vi "Logging Engine.vi"() -> ()   [LabVIEW 2016]
uses:
  <vilib>/DAQmx/read.llb/DAQmx Read (Analog Wfm 1Chan NSamp).vi
  <vilib>/TagLibrary/Create Tag (Int).vi
  <vilib>/TagLibrary/Write (Int).vi
  <vilib>/TagLibrary/Create Tag (String).vi
  <vilib>/TagLibrary/Write (String).vi
  <vilib>/TagLibrary/Write (Double).vi
  <vilib>/Message/Open (Sync).vi
  <vilib>/Message/Subscribe (Sync).vi
  <vilib>/DAQmx/miscellaneous.llb/DAQmx Fill In Error Info.vi
  <vilib>/Waveform/WDTOps.llb/WDT Number of Waveform Samples DBL.vi
  <vilib>/Waveform/WDTOps.llb/WDT Append Waveforms DBL.vi
  <vilib>/Message/Publish (Sync).vi
  <vilib>/TagLibrary/Read (Double).vi
  <vilib>/DAQmx/configure/timing.llb/DAQmx Timing (Sample Clock).vi
  <vilib>/TagLibrary/Read (Int).vi
  <vilib>/TagLibrary/Read (String).vi
  <vilib>/DAQmx/create/channels.llb/DAQmx Create Channel (AI-Temperature-Thermocouple).vi
  <vilib>/TagLibrary/Tag Library.lvlib
  <resource>/objmgr/niTag.rc
  <resource>/objmgr/daqmx.rc
panel:
  in  "Acquiring":bool
  out "Send Time":timestamp
  in  "Log":bool
  out "Status":string
  out "Channel":string
  out "error out":errorcluster
  out "Iteration":i32
  out "Waveform Channel":string
  in  "Send File":bool
  out "Sample Rate":dbl=1000.0 format="%0.2f"
  out "Files Sent":i32
  out "Buffered":i32
  in  "stop":bool
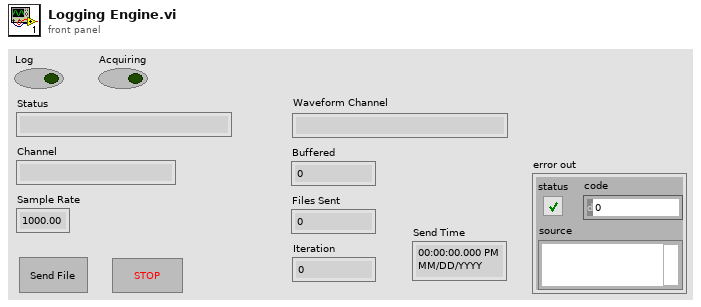
[diagram p1: front panel]
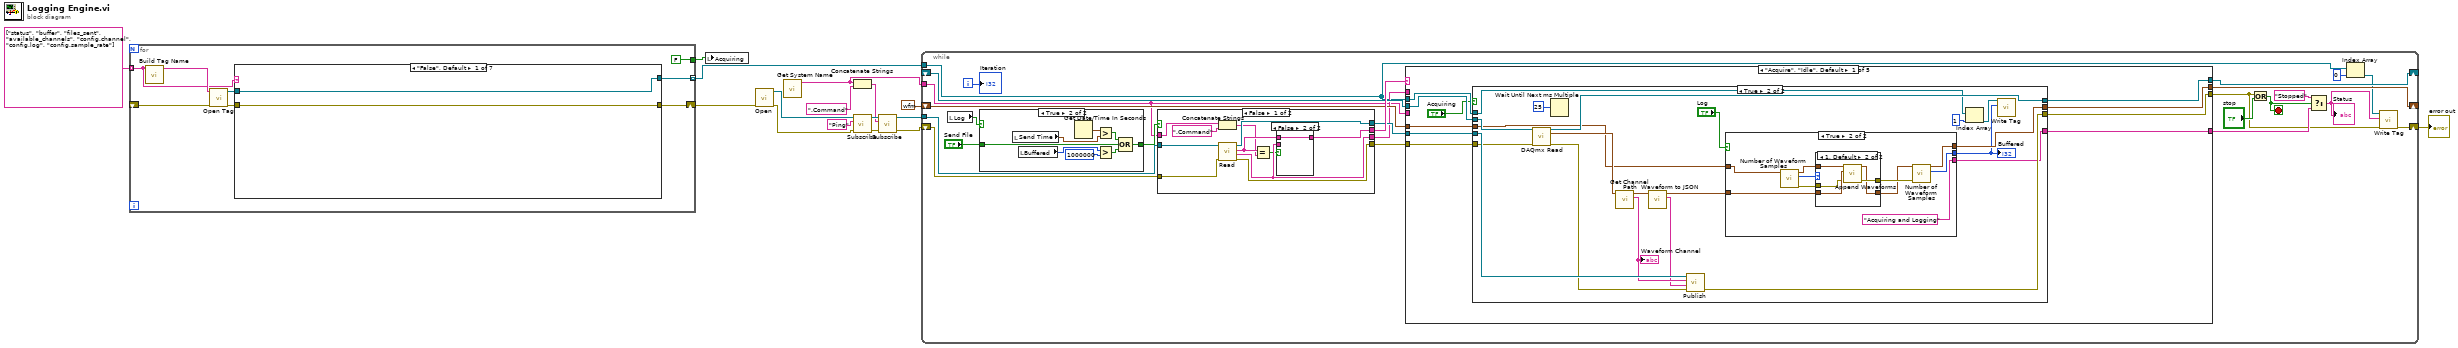
[diagram p0: block diagram]
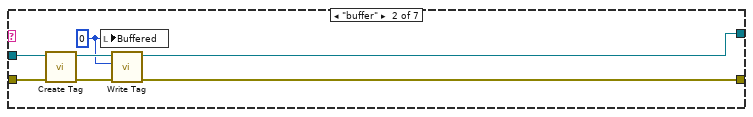
[diagram p2: hidden frame]
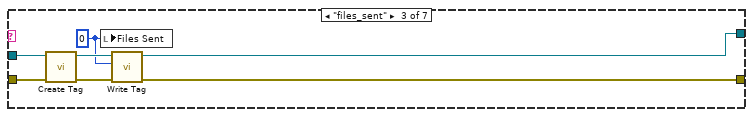
[diagram p3: hidden frame]
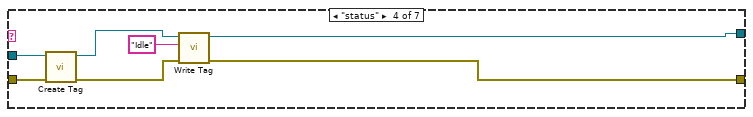
[diagram p4: hidden frame]
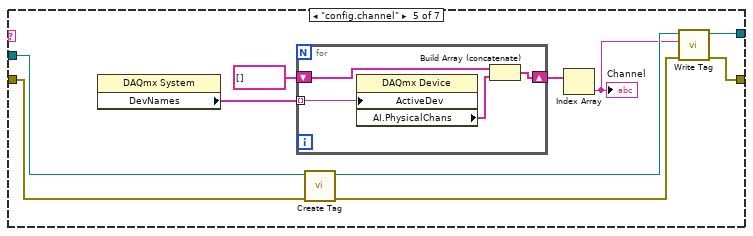
[diagram p5: hidden frame]
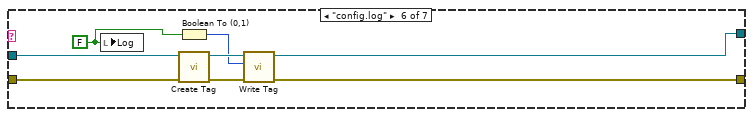
[diagram p6: hidden frame]
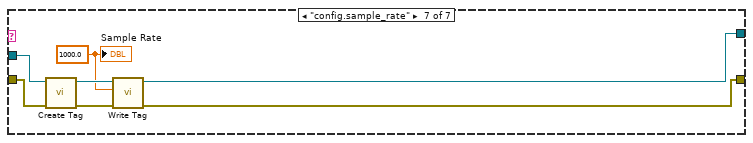
[diagram p7: hidden frame]
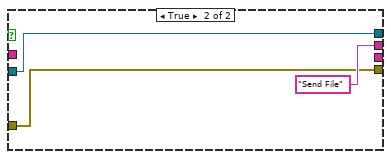
[diagram p10: hidden frame]
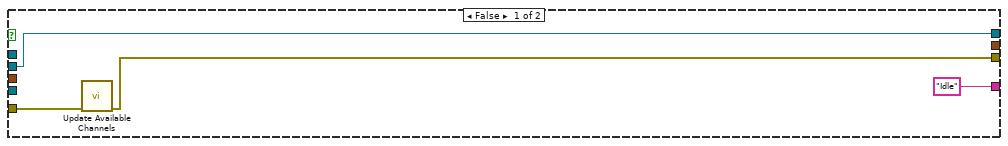
[diagram p11: hidden frame]
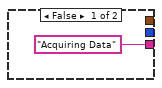
[diagram p12: hidden frame]
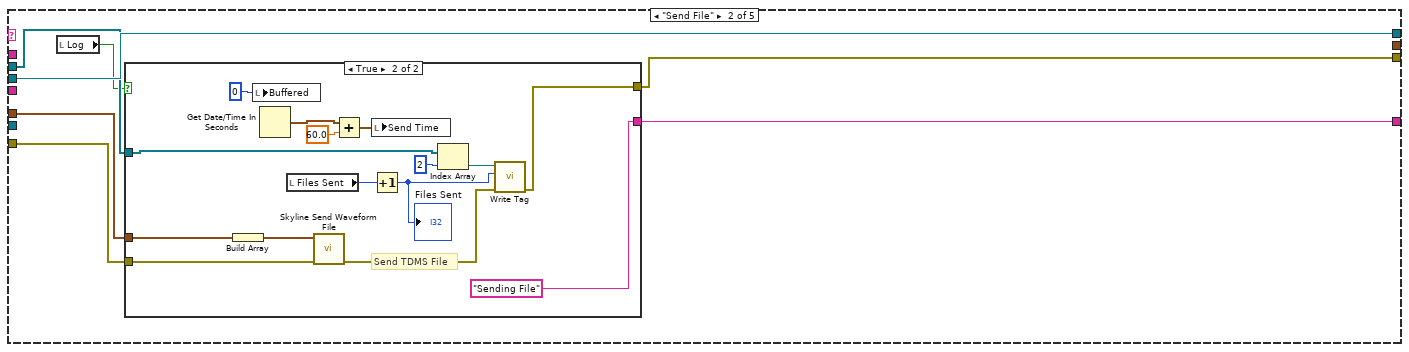
[diagram p14: hidden frame]
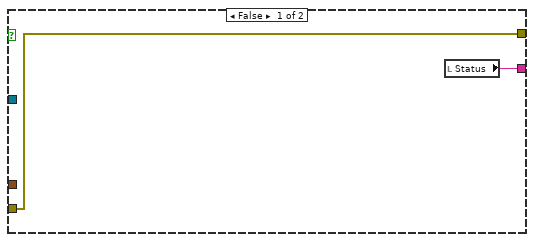
[diagram p15: hidden frame]
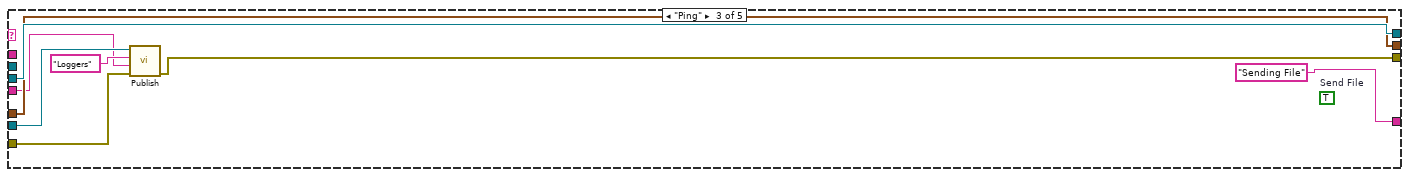
[diagram p16: hidden frame]
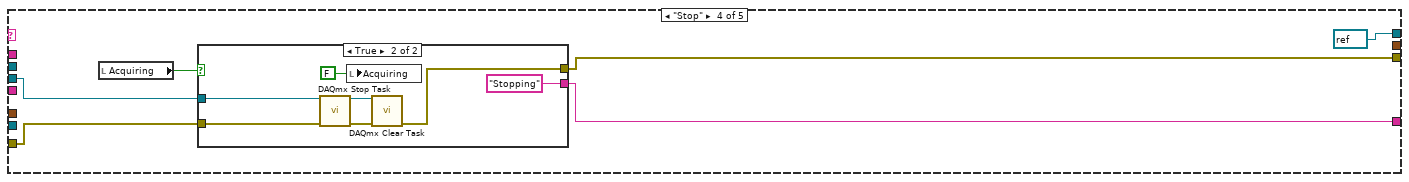
[diagram p17: hidden frame]
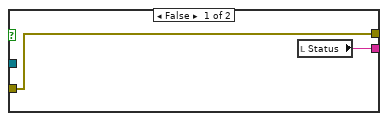
[diagram p18: hidden frame]
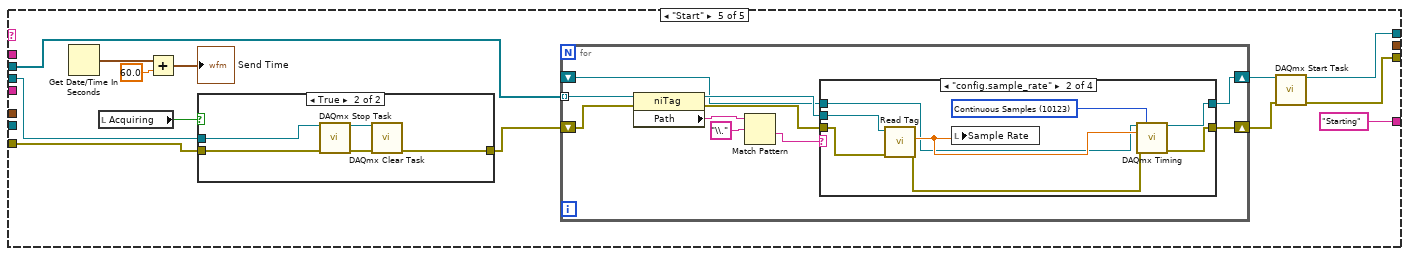
[diagram p19: hidden frame]
diagram:
  n1 = for {
    tunnel: [w23] -> w16 mode=indexing
    tunnel: string[] ["status", "buffer", "files_sent", "available_channels", "config.channel", "config.log", "config.sample_rate"] -> [w20] mode=indexing
    shift-right: [w19] -> w4
    shift-left: _ -> [w18]
    tunnel: [FALSE ("Acquiring")] -> w2
    n2 = call "Build Tag Name.vi"("Tag"=w20) -> ("System Tag"=w24:string)  [unwired: 10 in]
    n3 = call <vilib>:"Open Tag.vi"("error in (no error)"=w18, "tag path"=w24) -> ("error out"=w21:errorcluster, "tag reference out"=w22:refnum<k21>)  [unwired: 8 in]
    n4 = case shown="\"False\", Default" w20 {
      tunnel: [w25 w31 w38 w45 w53 w65 w72] -> w23
      tunnel: w22 -> [w25 w30 w37 w44 w57 w69 w76]
      tunnel: w21 -> [w26 w29 w36 w43 w56 w68 w75]
      tunnel: [w26 w28 w35 w41 w54 w66 w73] -> w19
      frame "False", Default {
      }
      frame "buffer" {
        w27 = 0 ("y")
        n5 = call-poly <vilib>:"Create Tag.vi"("error in (no error)"=w29, "tag reference in"=w30) -> ("error out"=w33:errorcluster, "tag reference out"=w32:refnum<k21>)  [unwired: 8 in]
        n6 = local write "Buffered"(w27) -> ()
        n7 = call-poly <vilib>:"Write Tag.vi"("error in (no error)"=w33, "int"=w27, "tag reference in"=w32) -> ("error out"=w28:errorcluster, "tag reference out"=w31:refnum<k21>)  [unwired: 7 in]
      }
      frame "files_sent" {
        w34 = 0 ("y")
        n8 = call-poly <vilib>:"Create Tag.vi"("error in (no error)"=w36, "tag reference in"=w37) -> ("error out"=w40:errorcluster, "tag reference out"=w39:refnum<k21>)  [unwired: 8 in]
        n9 = local write "Files Sent"(w34) -> ()
        n10 = call-poly <vilib>:"Write Tag.vi"("error in (no error)"=w40, "int"=w34, "tag reference in"=w39) -> ("error out"=w35:errorcluster, "tag reference out"=w38:refnum<k21>)  [unwired: 7 in]
      }
      frame "status" {
        n11 = call-poly <vilib>:"Create Tag.vi"("error in (no error)"=w43, "tag reference in"=w44) -> ("error out"=w47:errorcluster, "tag reference out"=w46:refnum<k21>)  [unwired: 8 in]
        n12 = call-poly <vilib>:"Write Tag.vi"("error in (no error)"=w47, "string"="Idle", "tag reference in"=w46) -> ("error out"=w41:errorcluster, "tag reference out"=w45:refnum<k21>)  [unwired: 7 in]
      }
      frame "config.channel" {
        n13 = property class="DAQmx System"() -> ("DevNames"=w51:tag[])  [unwired: 2 in, 2 out]
        n14 = for {
          tunnel: w51 -> [w61] mode=indexing
          shift-right: [w59] -> w49
          shift-left: string[] [] -> [w60]
          n15 = property class="DAQmx Device"("ActiveDev"=w61) -> ("AI.PhysicalChans"=w58:tag[])  [unwired: 2 in, 2 out]
          n16 = Build Array (concatenate)(w60, w58) -> (w59:string[])
        }
        n17 = call-poly <vilib>:"Create Tag.vi"("error in (no error)"=w56, "tag reference in"=w57) -> ("error out"=w52:errorcluster, "tag reference out"=w55:refnum<k21>)  [unwired: 8 in]
        n18 = Index Array(array=w49) -> (element=w48:string)  [unwired: 1 in]
        "Channel" <- w48
        n19 = call-poly <vilib>:"Write Tag.vi"("error in (no error)"=w52, "string"=w48, "tag reference in"=w55) -> ("error out"=w54:errorcluster, "tag reference out"=w53:refnum<k21>)  [unwired: 7 in]
      }
      frame "config.log" {
        w62 = FALSE ("Log")
        n20 = local write "Log"(w62) -> ()
        n21 = Boolean To (0,1)(Boolean=w62) -> (0, 1=w63:i16)
        n22 = call-poly <vilib>:"Create Tag.vi"("error in (no error)"=w68, "tag reference in"=w69) -> ("error out"=w64:errorcluster, "tag reference out"=w67:refnum<k21>)  [unwired: 8 in]
        n23 = call-poly <vilib>:"Write Tag.vi"("error in (no error)"=w64, "int"=w63, "tag reference in"=w67) -> ("error out"=w66:errorcluster, "tag reference out"=w65:refnum<k21>)  [unwired: 7 in]
      }
      frame "config.sample_rate" {
        w70 = 1000.0 ("double")
        n24 = call-poly <vilib>:"Create Tag.vi"("error in (no error)"=w75, "tag reference in"=w76) -> ("error out"=w71:errorcluster, "tag reference out"=w74:refnum<k21>)  [unwired: 8 in]
        n25 = call-poly <vilib>:"Write Tag.vi"("error in (no error)"=w71, "double"=w70, "tag reference in"=w74) -> ("error out"=w73:errorcluster, "tag reference out"=w72:refnum<k21>)  [unwired: 7 in]
        "Sample Rate" <- w70
      }
    }
  }
  n26 = local write "Acquiring"(w2) -> ()
  n27 = call-poly <vilib>:"Open.vi"("error in"=w4) -> ("error out"=w8:errorcluster, "Message Sync Refnum"=w9:refnum<k21>)  [unwired: 9 in]
  n28 = call "Get System Name.vi"() -> ("System Name"=w7:string)  [unwired: 11 in]
  n29 = Concatenate Strings(w7, ".Command" ("topic")) -> (w5:string)
  n30 = call-poly <vilib>:"Subscribe.vi"("error in (no error)"=w8, "topic"="Ping", "Message Sync Refnum"=w9) -> ("error out"=w11:errorcluster, "Message Sync Refnum"=w10:refnum<k21>)  [unwired: 7 in]
  n31 = call-poly <vilib>:"Subscribe.vi"("error in (no error)"=w11, "topic"=w5, "Message Sync Refnum"=w10) -> ("error out"=w13:errorcluster, "Message Sync Refnum"=w14:refnum<k21>)  [unwired: 7 in]
  n32 = while {
    shift-right: [w91] -> _
    shift-left: waveform(dbl) {"t0"=timestamp(0 s since 1904-01-01), "dt"=1.0, "Y"=[]} ("Waveform") -> [w93]
    tunnel: w16 -> [w89]
    tunnel: w14 -> [w97]
    shift-right: [w99] -> _
    shift-left: _ -> [w98]
    shift-right: [w81] -> w3
    shift-left: w13 -> [w96]
    tunnel: w7 -> [w86]
    i -> [w101]
    stop <- w84 stop-if-true
    n33 = local read "Log"() -> (w78:bool)
    n34 = case shown="True" w78 {
      tunnel: [_ w109] -> w90
      tunnel: "Send File" -> [_ w102]
      frame False {
      }
      frame True {
        n35 = local read "Send Time"() -> (w107:timestamp)
        n36 = local read "Buffered"() -> (w105:i32)
        n37 = Get Date/Time In Seconds() -> (seconds since 1Jan1904=w108:timestamp)
        n38 = Greater?(x=w108, y=w107) -> (0:w106:bool)
        n39 = Greater?(x=w105, y=1000000) -> (0:w104:bool)
        n40 = Compound Arithmetic op=OR(w106, w102, w104) -> (w109:bool)
      }
    }
    n41 = case shown="False" w90 {
      tunnel: [w116 "Send File" ("topic")] -> w100
      tunnel: w97 -> [w120 w124]
      tunnel: w96 -> [w119 w123]
      tunnel: [w118 w124] -> w95
      tunnel: [w117 w123] -> w94
      tunnel: [w115 _] -> w92
      tunnel: w86 -> [w111 _]
      frame False {
        n42 = Concatenate Strings(w111, ".Command" ("topic")) -> (w110:string)
        n43 = call <vilib>:"Read.vi"("error in (no error)"=w119, "Message Sync Refnum"=w120) -> ("error out"=w117:errorcluster, "message"=w115:string, "topic"=w113:string, "Message Sync Refnum"=w118:refnum<k21>)  [unwired: 5 in, 1 out]
        n44 = Equal?(x=w113, y=w110) -> (x = y?=w114:bool)
        n45 = case shown="False" w114 {
          tunnel: [w121 w122] -> w116
          tunnel: w115 -> [w121 _]
          tunnel: w113 -> [_ w122]
          frame True {
          }
          frame False {
          }
        }
      }
      frame True {
      }
    }
    n46 = case shown="\"Acquire\", \"Idle\", Default" w100 {
      tunnel: [w135 w184 w209 refnum<k21> refnum ("task out") w237] -> w99
      tunnel: w98 -> [w134 w184 w209 w215 w230]
      tunnel: w95 -> [w133 _ w204 _ _]
      tunnel: [w132 w179 w205 w214 w236] -> w80
      tunnel: w94 -> [w129 w182 w206 w213 w229]
      tunnel: [w131 _ w208 _ _] -> w91
      tunnel: w93 -> [w130 w181 w208 _ _]
      tunnel: w92 -> [_ _ _ _ _]
      tunnel: [w128 w183 "Sending File" w210 "Starting"] -> w83
      tunnel: w86 -> [_ _ w202 _ _]
      tunnel: w89 -> [w127 w180 _ _ w228]
      frame "Acquire", "Idle", Default {
        n47 = case shown="True" "Acquiring" {
          tunnel: [w139 w156] -> w135
          tunnel: w134 -> [w139 w155]
          tunnel: w133 -> [_ w154]
          tunnel: [w136 w150] -> w132
          tunnel: [_ w149] -> w131
          tunnel: w130 -> [_ w148]
          tunnel: w129 -> [w137 w147]
          tunnel: ["Idle" w146] -> w128
          tunnel: w127 -> [_ w144]
          frame False {
            n48 = call "Update Available Channels.vi"("error in (no error)"=w137) -> ("error out"=w136:errorcluster)  [unwired: 10 in]
          }
          frame True {
            n49 = call-poly <vilib>:"DAQmx Read.vi"("task/channels in"=w155, "error in"=w147) -> ("task out"=w156:refnum<k21>, "data"=w157:waveform(dbl), "error out"=w151:errorcluster)  [unwired: 11 in]
            n50 = Wait Until Next ms Multiple(millisecond multiple=u32 25) -> ()  [unwired: 1 out]
            n51 = call "Get Channel Path.vi"("Waveform"=w157) -> ("channel path"=w153:string, "Waveform out"=w158:waveform(dbl))  [unwired: 9 in]
            "Waveform Channel" <- w153
            n52 = call "Waveform to JSON.vi"("waveform in"=w158) -> ("JSON string"=w152:string, "waveform out"=w159:waveform(dbl))  [unwired: 9 in]
            n53 = call-poly <vilib>:"Publish.vi"("error in (no error)"=w151, "message"=w152, "topic"=w153, "Message Sync Refnum"=w154) -> ("error out"=w150:errorcluster)  [unwired: 6 in, 1 out]
            n54 = case shown="True" "Log" {
              tunnel: w159 -> [_ w168]
              tunnel: [_ w167] -> w149
              tunnel: w148 -> [_ w164]
              tunnel: [_ w166] -> w142
              tunnel: ["Acquiring Data" "Acquiring and Logging"] -> w146
              frame False {
              }
              frame True {
                n55 = call-poly <vilib>:"Number of Waveform Samples.vi"("waveform in"=w164) -> ("error out"=w162:errorcluster, "number of samples"=w163:i32, "waveform out"=w161:waveform(dbl))  [unwired: 8 in]
                n56 = case shown="1, Default" w163 {
                  tunnel: [w171 w177] -> w170
                  tunnel: [w172 w176] -> w169
                  tunnel: w168 -> [w172 w175]
                  tunnel: w161 -> [_ w174]
                  tunnel: w162 -> [w171 w173]
                  frame 0 {
                  }
                  frame 1, Default {
                    n57 = call-poly <vilib>:"Append Waveforms.vi"("error in (no error)"=w173, "waveform B"=w175, "waveform A"=w174) -> ("error out"=w177:errorcluster, "waveform out"=w176:waveform(dbl))  [unwired: 7 in]
                  }
                }
                n58 = call-poly <vilib>:"Number of Waveform Samples.vi"("error in (no error)"=w170, "waveform in"=w169) -> ("number of samples"=w166:i32, "waveform out"=w167:waveform(dbl))  [unwired: 7 in, 1 out]
              }
            }
            "Buffered" <- w142
            n59 = Index Array(array=w144, index=1) -> (element=w143:refnum<k21>)
            n60 = call-poly <vilib>:"Write Tag.vi"("int"=w142, "tag reference in"=w143) -> ()  [unwired: 8 in, 2 out]
          }
        }
      }
      frame "Send File" {
        n61 = local read "Log"() -> (w178:bool)
        n62 = case shown="True" w178 {
          tunnel: [w186 "Sending File"] -> w183
          tunnel: w182 -> [w185 w198]
          tunnel: w181 -> [_ w197]
          tunnel: w180 -> [_ w196]
          tunnel: [w185 w193] -> w179
          frame False {
            n63 = local read "Status"() -> (w186:string)
          }
          frame True {
            # "Send TDMS File"
            n64 = Build Array(w197) -> (w199:waveform(dbl)[])
            n65 = local write "Buffered"(0 ("Buffered")) -> ()
            n66 = Get Date/Time In Seconds() -> (seconds since 1Jan1904=w191:timestamp)
            n67 = local read "Files Sent"() -> (w194:i32)
            n68 = call "Skyline Send Waveform File.vi"("error in"=w198, "data in"=w199) -> ("error out"=w200:errorcluster)  [unwired: 7 in, 2 out]
            n69 = Add(x=w191, y=60.0) -> (x+y=w192:timestamp)
            n70 = local write "Send Time"(w192) -> ()
            n71 = Increment(x=w194) -> (x+1=w195:i32)
            "Files Sent" <- w195
            n72 = Index Array(array=w196, index=2) -> (element=w187:refnum<k21>)
            n73 = call-poly <vilib>:"Write Tag.vi"("error in (no error)"=w200, "int"=w195, "tag reference in"=w187) -> ("error out"=w193:errorcluster)  [unwired: 7 in, 1 out]
          }
        }
      }
      frame "Ping" {
        (unwired) TRUE  # Send File
        n74 = call-poly <vilib>:"Publish.vi"("error in (no error)"=w206, "message"=w202, "topic"="Loggers", "Message Sync Refnum"=w204) -> ("error out"=w205:errorcluster)  [unwired: 6 in, 1 out]
      }
      frame "Stop" {
        n75 = local read "Acquiring"() -> (w211:bool)
        n76 = case shown="True" w211 {
          tunnel: w215 -> [_ w222]
          tunnel: [w217 w221] -> w214
          tunnel: w213 -> [w217 w220]
          tunnel: [w216 "Stopping"] -> w210
          frame False {
            n77 = local read "Status"() -> (w216:string)
          }
          frame True {
            n78 = call <vilib>:"DAQmx Stop Task.vi"("task/channels in"=w222, "error in"=w220) -> ("task out"=w224:refnum<k21>, "error out"=w223:errorcluster)  [unwired: 12 in]
            n79 = local write "Acquiring"(FALSE ("Acquiring")) -> ()
            n80 = call <vilib>:"DAQmx Clear Task.vi"("task in"=w224, "error in"=w223) -> ("error out"=w221:errorcluster)  [unwired: 13 in]
          }
        }
      }
      frame "Start" {
        n81 = Get Date/Time In Seconds() -> (seconds since 1Jan1904=w233:timestamp)
        n82 = local read "Acquiring"() -> (w231:bool)
        n83 = Add(x=w233, y=60.0) -> (x+y=→"Send Time":timestamp)
        n84 = case shown="True" w231 {
          tunnel: w230 -> [_ w275]
          tunnel: w229 -> [w272 w274]
          tunnel: [w272 w273] -> w227
          frame False {
            n85 = local write "Acquiring"(TRUE ("Running")) -> ()
          }
          frame True {
            n86 = call <vilib>:"DAQmx Stop Task.vi"("task/channels in"=w275, "error in"=w274) -> ("task out"=w277:refnum<k21>, "error out"=w276:errorcluster)  [unwired: 12 in]
            n87 = call <vilib>:"DAQmx Clear Task.vi"("task in"=w277, "error in"=w276) -> ("error out"=w273:errorcluster)  [unwired: 13 in]
          }
        }
        n88 = for {
          tunnel: w228 -> [w247] mode=indexing
          shift-right: [w241] -> w226
          shift-left: w227 -> [w243]
          shift-right: [w239] -> w225
          shift-left: _ -> [w238]
          n89 = property class="niTag"(reference=w247, error in=w243) -> (reference out=w242:refnum<k21>, error out=w240:errorcluster, "Path"=w246:string)
          n90 = Match Pattern(string=w246, regular expression="\\.") -> (after substring=w244:string)  [unwired: 1 in, 3 out]
          n91 = case shown="\"config.sample_rate\"" w244 {
            tunnel: w242 -> [_ w255 w264 w270]
            tunnel: [w249 w254 w262 w268] -> w241
            tunnel: w240 -> [w249 w253 w263 w269]
            tunnel: [w248 w250 w258 w265] -> w239
            tunnel: w238 -> [w248 w251 w258 _]
            frame "False", Default {
            }
            frame "config.sample_rate" {
              w257 = 10123 items=["Finite Samples"=10178, "Continuous Samples"=10123, "Hardware Timed Single Point"=12522] ("sample mode")
              n92 = call-poly <vilib>:"Read Tag.vi"("error in (no error)"=w253, "tag reference in"=w255) -> ("error out"=w256:errorcluster, "double"=w252:dbl)  [unwired: 5 in, 3 out]
              n93 = local write "Sample Rate"(w252) -> ()
              n94 = call-poly <vilib>:"DAQmx Timing.vi"("task/channels in"=w251, "sample mode"=w257, "rate"=w252, "error in"=w256) -> ("task out"=w250:refnum<k21>, "error out"=w254:errorcluster)  [unwired: 10 in]
            }
            frame "config.log" {
              n95 = call-poly <vilib>:"Read Tag.vi"("error in (no error)"=w263, "tag reference in"=w264) -> ("error out"=w262:errorcluster, "integer"=w261:i32)  [unwired: 5 in, 3 out]
              n96 = Number To Boolean Array(number=w261) -> (Boolean array=w260:bool[])
              n97 = Index Array(array=w260) -> (element=w259:bool)  [unwired: 1 in]
              n98 = local write "Log"(w259) -> ()
            }
            frame "config.channel" {
              n99 = call-poly <vilib>:"Read Tag.vi"("error in (no error)"=w269, "tag reference in"=w270) -> ("error out"=w267:errorcluster, "string"=w266:string)  [unwired: 6 in, 2 out]
              n100 = local write "Channel"(w266) -> ()
              n101 = call-poly <vilib>:"DAQmx Create Virtual Channel.vi"("physical channels"=w266, "error in"=w267) -> ("task out"=w265:refnum<k21>, "error out"=w268:errorcluster)  [unwired: 12 in]
            }
          }
        }
        n102 = call <vilib>:"DAQmx Start Task.vi"("task/channels in"=w225, "error in"=w226) -> ("task out"=w237:refnum<k21>, "error out"=w236:errorcluster)  [unwired: 12 in]
      }
    }
    n103 = Or(x=w80, y="stop") -> (x .or. y?=w84:bool)
    n104 = Select(t="Stopped", s=w84, f=w83) -> (s? t:f=w79:string)
    "Status" <- w79
    n105 = Index Array(array=w89, index=0) -> (element=w87:refnum<k21>)
    n106 = call-poly <vilib>:"Write Tag.vi"("error in (no error)"=w80, "string"=w79, "tag reference in"=w87) -> ("error out"=w81:errorcluster)  [unwired: 7 in, 1 out]
    "Iteration" <- w101
  }
  "error out" <- w3
